vi "XNET.DB.Initialize.vi"(8 "error in (no error)":errorcluster, 11 "Parameters":T1={"Name"="", "CAN"={"Interface"="", "Baud Rate"=0, "Diagnostic Protocol"=enum."GMLAN", "Transport Protocol"=enum."ISO TP - Normal Mode", "Transmit ID"=0, "Receive ID"=2, "Transmit Extension"=1, "Receive Extension"=255, "Receive UUDT ID"=0, "Enable Stream"=TRUE, "VW TP Channel ID"=1, "Fill Frame"=FALSE, "Fill Byte"=0, "Termination"=FALSE, "LIN Cluster"="", "NAD"=8, "IO Mode"=0, "Max DLC"=0, "FD Baud Rate"=2, "Timeout"=1, "FD ISO Mode"=0, "DoIP Address"="", "DoIP Source Address"=3584, "DoIP Dynamic Port"=TRUE, "DoIP Version"=2}, "986x"={"Enable"=FALSE, "RIO Device"="", "Bitfile"=path ""}, "Reads"=[], "Frames Lookup"=variant(enum16{"GMLAN", "KWP-2000", "UDS"} enum."GMLAN"), "Writes"=[], "DPIDs"=[], "DPID Lookup"=variant(u32 0), "DTC"={"Descriptor"={"DTC Byte Length"=1, "Status Byte Length"=1, "Add Data Byte Length"=1, "Byte Order"=enum."Motorola"}, "Value.Code"=[], "Value.String"=[], "Value.J2012String"=[], "Status.Code"=[], "Status.String"=[]}, "Created DTCs"=0, "Polls"=[], "Service Channels Status Lookup"=variant, "Trigger Lookup"=variant, "Security"={"Type"=enum."None", "Source DLL Path"=path "", "Target DLL Path"=path "", "Security Level"=0}} {"Writes"."Signals"."Byte Order" items=["Little Endian", "Big Endian"]; "Writes"."Signals"."Data Type" items=["Signed", "Unsigned", "IEEE Float"]; "CAN"."DoIP Version" items=["2010"=1, "2012"=2]; "CAN"."DoIP Source Address" format="%.0x"; "CAN"."FD ISO Mode" items=["ISO", "Non ISO", "ISO Legacy"]; "CAN"."IO Mode" items=["CAN 2.0", "CAN FD", "CAN FD+BRS"]; "CAN"."Fill Byte" format="%.0x"; "CAN"."VW TP Channel ID" format="%.0x"; "CAN"."Receive UUDT ID" format="%.0x"; "CAN"."Receive Extension" format="%.0x"; "CAN"."Transmit Extension" format="%.0x"; "CAN"."Receive ID" format="%.0x"; "CAN"."Transmit ID" format="%.0x"; "Reads"."Signals"."Byte Order" items=["Little Endian", "Big Endian"]; "Reads"."Signals"."Data Type" items=["Signed", "Unsigned", "IEEE Float"]}) -> (0 "error out":errorcluster, 2 "Convert Session Cluster":refnum<k21>, 3 "XNET Database":refnum<k21>)   [LabVIEW 2019, in "Diagnostics Addon Engine.lvlib"]
uses:
  Diagnostics Addon Engine.lvlib
  Addon Shared/Types/SysDef.Compile.ctl
  Addon Shared/Types/CAN.ctl
  Addon Shared/Types/CAN.Interface.ctl
  Addon Shared/Types/Protocol.ctl
  Addon Shared/Types/Transport.ctl
  Addon Shared/Types/986x.ctl
  Addon Shared/Types/Frame.Compile.ctl
  Addon Shared/Types/Type.ctl
  Addon Shared/Types/Signal.ctl
  Addon Shared/Types/DPID.ctl
  Addon Shared/Types/DPID.Rate.ctl
  Addon Shared/Types/DTC.Settings.ctl
  Addon Shared/Types/DTC.Descriptor.ctl
  Addon Shared/Types/Poll.Compiled.ctl
  Addon Shared/Types/Security.ctl
  Addon Shared/Types/Security.Type.ctl
  Types/XNET.Cluster.ctl
  <vilib>/xnet/xnet.llb/XNET Database Open (Database).vi
  <resource>/objmgr/xnet.rc
  Addon Shared/Diagnostics Addon Shared.lvlib
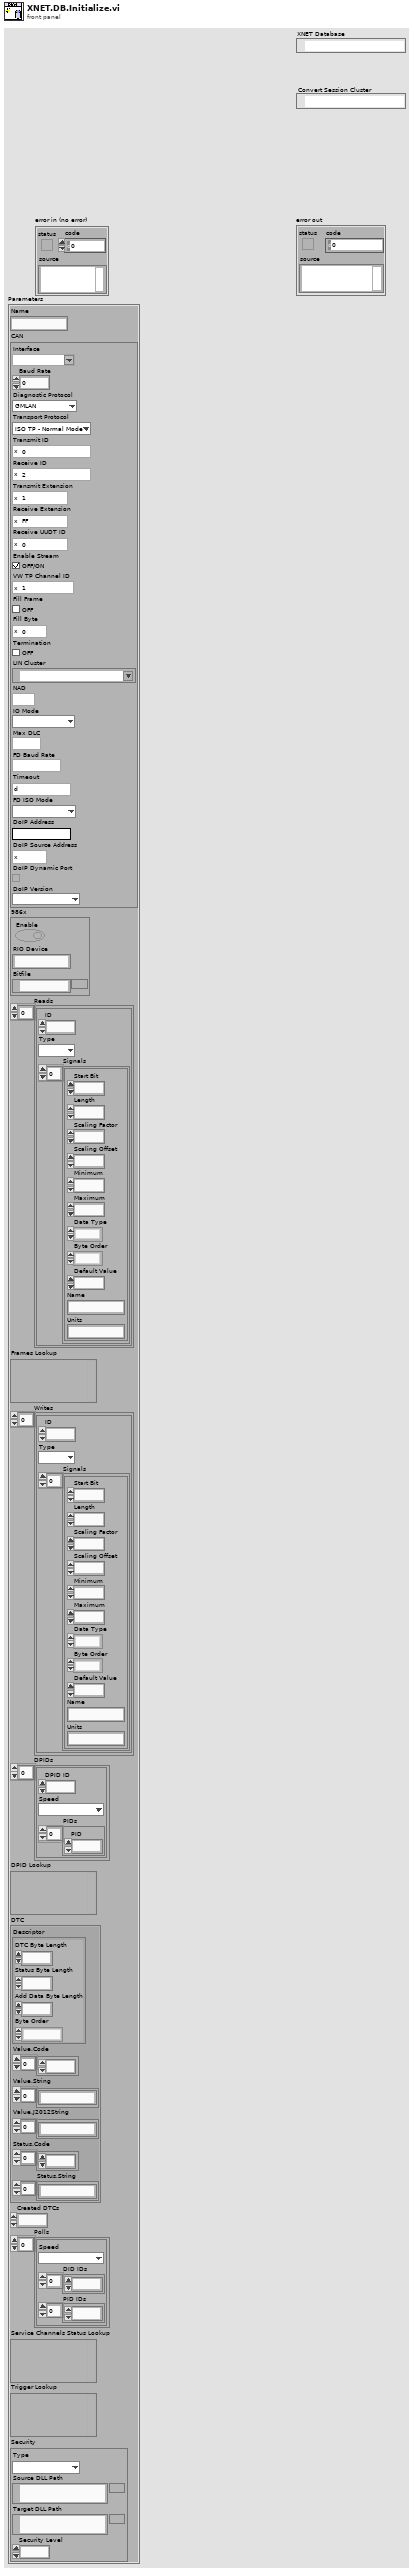
[diagram p1: front panel]
types:
  T1 = typedef "Diagnostics Addon Shared.lvlib/SysDef.Compile.ctl" = cluster{"Name":string, "CAN":T2, "986x":T6, "Reads":T7[], "Frames Lookup":variant, "Writes":T7[], "DPIDs":T10[], "DPID Lookup":variant, "DTC":T12, "Created DTCs":u32, "Polls":T14[], "Service Channels Status Lookup":variant, "Trigger Lookup":variant, "Security":T15}
  T2 = typedef "Diagnostics Addon Shared.lvlib/CAN.ctl" = cluster{"Interface":T3, "Baud Rate":u64, "Diagnostic Protocol":T4, "Transport Protocol":T5, "Transmit ID":u32, "Receive ID":u32, "Transmit Extension":u8, "Receive Extension":u8, "Receive UUDT ID":u32, "Enable Stream":bool, "VW TP Channel ID":u32, "Fill Frame":bool, "Fill Byte":u8, "Termination":bool, "LIN Cluster":refnum<k21>, "NAD":u8, "IO Mode":u32, "Max DLC":u16, "FD Baud Rate":u64, "Timeout":u32, "FD ISO Mode":u32, "DoIP Address":string, "DoIP Source Address":u16, "DoIP Dynamic Port":bool, "DoIP Version":u16}
  T3 = typedef "Diagnostics Addon Shared.lvlib/CAN.Interface.ctl" = string
  T4 = typedef "Diagnostics Addon Shared.lvlib/Protocol.ctl" = enum16{"GMLAN", "KWP-2000", "UDS", "User-Defined"}
  T5 = typedef "Diagnostics Addon Shared.lvlib/Transport.ctl" = enum16{"ISO TP - Normal Mode", "ISO TP - Mixed Mode", "VW TP 2.0", "Diagnostics on IP", "ISO TP LIN"}
  T6 = typedef "Diagnostics Addon Shared.lvlib/986x.ctl" = cluster{"Enable":bool, "RIO Device":string, "Bitfile":path}
  T7 = typedef "Diagnostics Addon Shared.lvlib/Frame.Compile.ctl" = cluster{"ID":u32, "Type":T8, "Signals":T9[]}
  T8 = typedef "Diagnostics Addon Shared.lvlib/Type.ctl" = enum16{"DID", "CDID", "PID", "CPID", "Read Memory", "Write Memory", "IO Control", "Routine Start", "Routine Request", "Routine Stop", "User Defined", "DTC Control", "Clear DTCs", "Read DTCs", "Start DTCs", "DTC Change Count", "Tester Present", "Unlock ECU", "Reset ECU", "Diag Session Control", "Communication Control", "DPID Control", "Poll Control", "Diag CAN Control"}
  T9 = typedef "Diagnostics Addon Shared.lvlib/Signal.ctl" = cluster{"Start Bit":u32, "Length":u32, "Scaling Factor":dbl, "Scaling Offset":dbl, "Minimum":dbl, "Maximum":dbl, "Data Type":u32, "Byte Order":u32, "Default Value":dbl, "Name":string, "Units":string}
  T10 = typedef "Diagnostics Addon Shared.lvlib/DPID.ctl" = cluster{"DPID ID":u8, "Speed":T11, "PIDs":u16[]}
  T11 = typedef "Diagnostics Addon Shared.lvlib/DPID.Rate.ctl" = enum16{"Slow", "Medium", "Fast"}
  T12 = typedef "Diagnostics Addon Shared.lvlib/DTC.Settings.ctl" = cluster{"Descriptor":T13, "Value.Code":dbl[], "Value.String":string[], "Value.J2012String":string[], "Status.Code":dbl[], "Status.String":string[]}
  T13 = typedef "Diagnostics Addon Shared.lvlib/DTC.Descriptor.ctl" = cluster{"DTC Byte Length":i32, "Status Byte Length":i32, "Add Data Byte Length":i32, "Byte Order":enum16{"Motorola", "Intel"}}
  T14 = typedef "Diagnostics Addon Shared.lvlib/Poll.Compiled.ctl" = cluster{"Speed":T11, "DID IDs":u32[], "PID IDs":u32[]}
  T15 = typedef "Diagnostics Addon Shared.lvlib/Security.ctl" = cluster{"Type":T16, "Source DLL Path":path, "Target DLL Path":path, "Security Level":u8}
  T16 = typedef "Diagnostics Addon Shared.lvlib/Security.Type.ctl" = enum16{"None", "SeedKey", "MasterKey"}
  T17 = typedef "Diagnostics Addon Engine.lvlib/XNET.Cluster.ctl" = cluster{"64bit Baud Rate":u64, "Comment":string, "Name":string, "Transmit I/O Mode":u32, "64bit FD Baud Rate":u64}
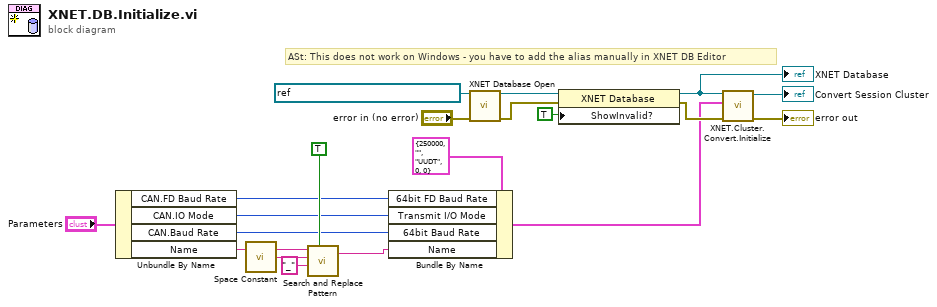
[diagram p0: block diagram]
diagram:
  # "ASt: This does not work on Windows - you have to add the alias manually in XNET DB Editor"
  n1 = Unbundle By Name("Parameters") -> ("CAN.FD Baud Rate"=w5:u64, "CAN.IO Mode"=w6:u32, "CAN.Baud Rate"=w7:u64, "Name"=w8:string)
  n2 = call <vilib>:"Space Constant.vi"() -> ("String"=w17:string)
  n3 = call <vilib>:"Search and Replace Pattern.vi"("string"=w8, "regular expression (\"\")"=w17, "replace string (\"\")"="_" ("replace string (\"\")"), "replace all? (F)"=TRUE) -> ("result string"=w16:string)  [unwired: 1 in, 1 out]
  n4 = Bundle By Name(cluster=T17 {"64bit Baud Rate"=250000, "Comment"="", "Name"="UUDT", "Transmit I/O Mode"=0, "64bit FD Baud Rate"=0} ("CAN Cluster"), "64bit FD Baud Rate"=w5, "Transmit I/O Mode"=w6, "64bit Baud Rate"=w7, "Name"=w16) -> (w4:T17)
  n5 = call-poly <vilib>:"XNET Database Open.vi"("database in (:memory:)"=refnum<k21> "Diagnostics_Addon_Temp_DB", "error in (no error)"="error in (no error)") -> ("database out"=w11:refnum<k21>, "error out"=w15:errorcluster)  [unwired: 12 out]
  n6 = property class="XNET Database"(reference=w11, error in=w15, "ShowInvalid?"=TRUE ("Show Invalid From Open?")) -> (reference out=w2:refnum<k21>, error out=w14:errorcluster)
  "XNET Database" <- w2
  n7 = call "XNET.Cluster.Convert.Initialize.vi"("error in"=w14, "CAN Cluster"=w4, "database in"=w2) -> ("error out"=→"error out":errorcluster, "cluster out"=→"Convert Session Cluster":refnum<k21>)  [unwired: 7 out]
